vi "Get Events.vi"(11 "Create Sensor View in":refnum<class "Edit Sensor View.lvclass">) -> (2 "Events":T1, 3 "Create Sensor View out":refnum<class "Edit Sensor View.lvclass">)   [LabVIEW 2013, in "Edit Sensor View.lvlib" / "Edit Sensor View.lvclass"]
uses:
  Edit Sensor View.lvclass
  Typedef/Events.ctl
  Edit Sensor View.lvclass/Edit Sensor View.ctl
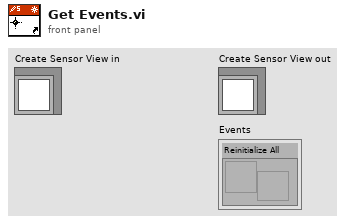
[diagram p1: front panel]
types:
  T1 = typedef "Edit Sensor View.lvlib/Edit Sensor View.lvclass/Events.ctl" = cluster{"Reinitialize All":refnum<user-event>}
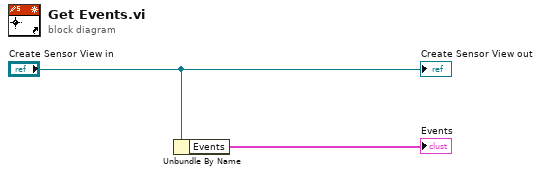
[diagram p0: block diagram]
diagram:
  n1 = Unbundle By Name("Create Sensor View in") -> ("Events"=→"Events":T1)
  "Create Sensor View out" <- "Create Sensor View in"
